vi "CloseConnection.vi"(8 "error in (no error)":errorcluster, 11 "TCP_Server_Connection_Handler in":refnum<class "TCP_Server_Connection_Handler.lvclass">) -> (0 "error out":errorcluster, 3 "TCP_Server_Connection_Handler out":refnum<class "TCP_Server_Connection_Handler.lvclass">)   [LabVIEW 2023, in "TCP_Server_Connection_Handler.lvlib" / "TCP_Server_Connection_Handler.lvclass"]
uses:
  TCP_Server_Connection_Handler.lvclass
  TCP_Server_Connection_Handler.lvclass/TCP_Server_Connection_Handler.ctl
  TCP_Server_Connection_Handler Messages/SendString Msg/SendString Msg.lvclass
  <vilib>/ActorFramework/Actor/Actor.lvclass
  <vilib>/ActorFramework/Stop Msg/Stop Msg.lvclass
  C:/Program Files (x86)/National Instruments/LabVIEW 2023/vi.lib/ActorFramework/Actor/Actor.lvclass
  C:/Source/LabVIEW/TCP_server/TCP_Server_Connection_Handler/TCP_Server_Connection_Handler/TCP_Server_Connection_Handler.lvclass
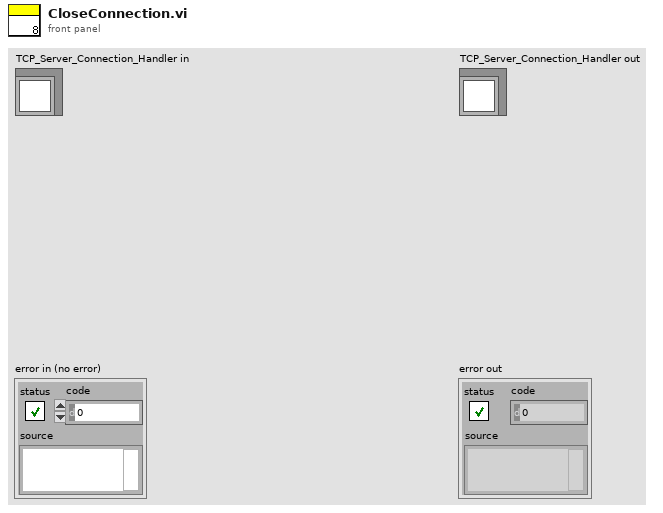
[diagram p1: front panel]
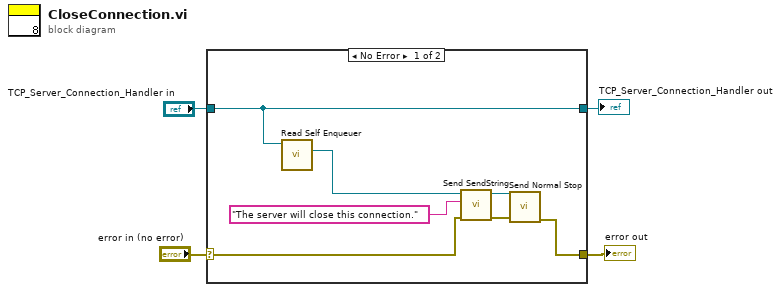
[diagram p0: block diagram]
diagram:
  n1 = case shown="No Error" "error in (no error)" {
    selector: "error in (no error)" -> [w6 w13]
    tunnel: [w5 w13] -> w3
    tunnel: [w11 w12] -> w1
    tunnel: "TCP_Server_Connection_Handler in" -> [w11 w12]
    frame No Error {
      n2 = call <vilib>:"Read Self Enqueuer.vi"("Actor"=w11) -> ("Self Enqueuer"=w10:refnum<class "Message Enqueuer.lvclass">)  [unwired: 10 in]
      n3 = call "Send SendString.vi"("error in (no error)"=w6, "Message"="The server will close this connection.", "Message Enqueuer"=w10) -> ("error out"=w8:errorcluster, "Message Enqueuer out"=w7:refnum<class "Message Enqueuer.lvclass">)  [unwired: 7 in]
      n4 = call <vilib>:"Send Normal Stop.vi"("error in (no error)"=w8, "Message Enqueuer"=w7) -> ("error out"=w5:errorcluster)  [unwired: 9 in]
    }
    frame Error {
    }
  }
  "error out" <- w3
  "TCP_Server_Connection_Handler out" <- w1
